vi "4-element-Linearization.vi"(1 "B":i32, 2 "Voltage in":dbl, 3 "C4":i32, 4 "C3":i32, 5 "C2":i32, 6 "C1":i32) -> (0 "Scaled value":dbl)   [LabVIEW 2020]
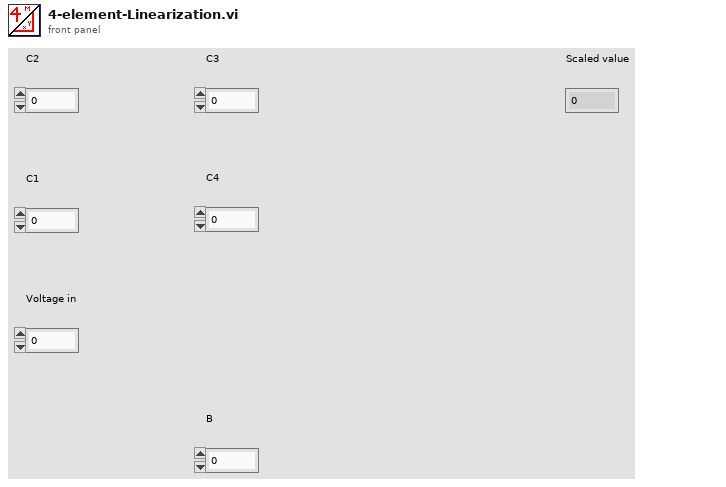
[diagram p1: front panel]
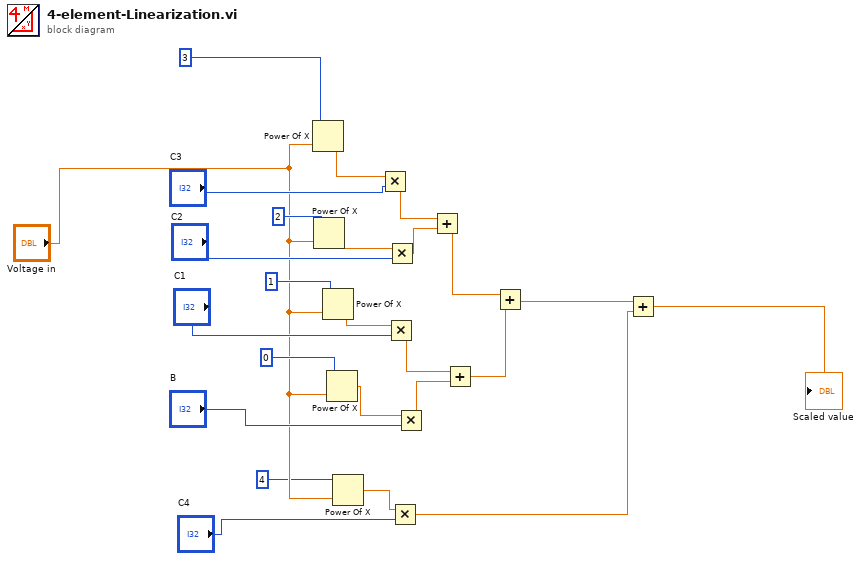
[diagram p0: block diagram]
diagram:
  n1 = Power Of X(1:"Voltage in", 2:3) -> (0:w10:dbl)
  n2 = Power Of X(1:"Voltage in", 2:2) -> (0:w14:dbl)
  n3 = Power Of X(1:"Voltage in", 2:1) -> (0:w16:dbl)
  n4 = Power Of X(1:"Voltage in", 2:0) -> (0:w18:dbl)
  n5 = Power Of X(1:"Voltage in", 2:4) -> (0:w6:dbl)
  n6 = Multiply(x=w10, y="C3") -> (x*y=w21:dbl)
  n7 = Multiply(x=w16, y="C1") -> (x*y=w23:dbl)
  n8 = Multiply(x=w14, y="C2") -> (x*y=w20:dbl)
  n9 = Multiply(x=w6, y="C4") -> (x*y=w2:dbl)
  n10 = Multiply(x=w18, y="B") -> (x*y=w22:dbl)
  n11 = Add(x=w21, y=w20) -> (x+y=w25:dbl)
  n12 = Add(x=w23, y=w22) -> (x+y=w24:dbl)
  n13 = Add(x=w25, y=w24) -> (x+y=w4:dbl)
  n14 = Add(x=w4, y=w2) -> (x+y=→"Scaled value":dbl)
